vi "Get Connector Pane Info.vi"(8 "error in (no error)":errorcluster, 11 "vi reference":refnum<vi>) -> (0 "error out":errorcluster, 3 "Terminals":T1[](array[typedef]))   [LabVIEW 2025, in "MCP Server.lvlib"]
doc: "Utilizes the Application method \"Get ConPane Datatype\" to read the terminal properties of a subVI without loading it or requiring VI scripting."
uses:
  MCP Server.lvlib
  Terminal.ctl
  <vilib>/Utility/Data Type/NI_Data Type.lvlib
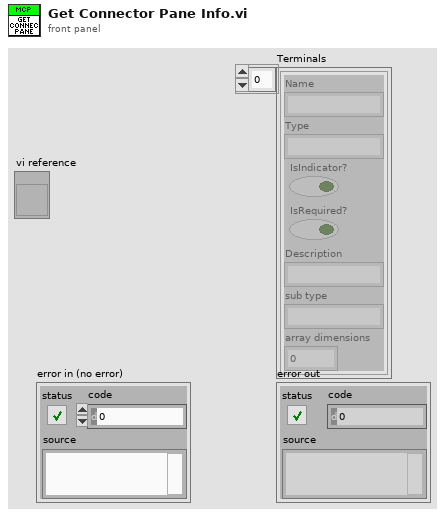
[diagram p1: front panel]
types:
  T1 = typedef "MCP Server.lvlib/Terminal.ctl" = cluster{"Name":string, "Type":string, "IsIndicator?":bool, "IsRequired?":bool, "Description":string, "sub type":string, "array dimensions":i32}
  T2 = typedef "NI_Data Type.lvlib/VI Info.ctl" = cluster{"Connector Pane Pattern":i16, "Connector Pane Rotation":i16, "Flags":u32[], "Modification Date":timestamp, "Asynchronous":bool, "Non-Function":bool, "Subroutine":bool, "SubSystem":bool}
  T3 = typedef "NI_Data Type.lvlib/Data Type.ctl" = enum8{"Invalid Type", "Void", "I8", "I16", "I32", "I64", "U8", "U16", "U32", "U64", "Single Float", "Double Float", "Extended Float", "Single Complex", "Double Complex", "Extended Complex", "Enum U8", "Enum U16", "Enum U32", "Enum U64", "Single Float With Unit", "Double Float With Unit", "Extended Float With Unit", "Single Complex with Unit", "Double Complex with Unit", "Extended Complex with Unit", "Boolean", "String", "Path", "Picture", "Tag", "Array", "Cluster", "Variant", "LV Variant", "Waveform", "Timestamp", "Digital Waveform", "Digital Data", "ExpressData", "Refnum", "External Data", "VI", "Poly VI", "LabVIEW Class Instance", "Fixed Point", "Set Collection", "Map Collection"}
  T4 = typedef "NI_Data Type.lvlib/Memory Info.ctl" = cluster{"Type":T5, "Size":u32}
  T5 = typedef "NI_Data Type.lvlib/Memory Type.ctl" = enum16{"Variable", "Fixed", "Bounded"}
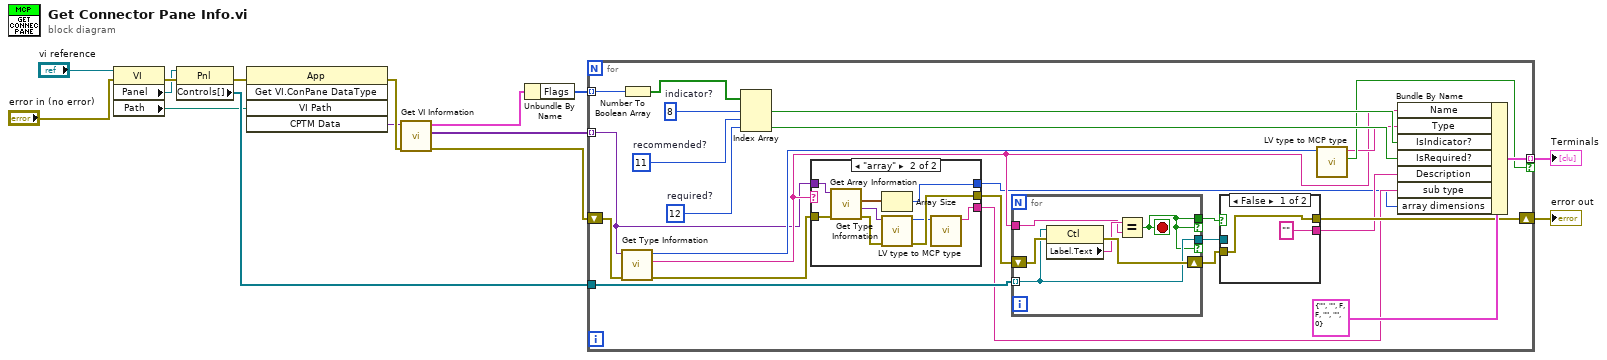
[diagram p0: block diagram]
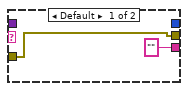
[diagram p2: hidden frame]
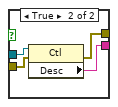
[diagram p3: hidden frame]
diagram:
  n1 = property class="VI"(reference="vi reference", error in="error in (no error)") -> (error out=w6:errorcluster, "Panel"=w4:refnum<vi>, "Path"=w1:path)  [unwired: 1 out]
  n2 = property class="Pnl"(reference=w4, error in=w6) -> (error out=w5:errorcluster, "Controls[]"=w3:refnum<vi>[])  [unwired: 1 out]
  n3 = invoke class="App" method="Get VI.ConPane DataType"(error in=w5, "VI Path"=w1) -> (error out=w12:errorcluster, "CPTM Data"=w8:variant)  [unwired: 3 in, 3 out]
  n4 = call <vilib>:"Get VI Information.vi"("error in (no error)"=w12, "variant"=w8) -> ("error out"=w11:errorcluster, "VI terminal types"=w7:variant[], "VI info"=w9:T2)  [unwired: 6 in, 1 out]
  n5 = Unbundle By Name(w9) -> ("Flags"=w10:u32[])
  n6 = for {
    tunnel: w7 -> [w18] mode=indexing
    tunnel: w10 -> [w39] mode=indexing
    shift-right: [w24] -> w14
    shift-left: w11 -> [w33]
    tunnel: [w29] -> w15 mode=indexing if=w28
    tunnel: w3 -> [w25]
    w35 = 12  # required?
    w36 = 11  # recommended?
    w37 = 8  # indicator?
    n7 = call <vilib>:"Get Type Information.vi"("error in (no error)"=w33, "variant"=w18) -> ("error out"=w34:errorcluster, "name"=w19:string, "type"=w40:T3)  [unwired: 5 in, 2 out]
    n8 = Number To Boolean Array(number=w39) -> (Boolean array=w38:bool[])
    n9 = Index Array(array=w38, index #1=w37, index #2=w36, index #3=w35) -> (element #1=w31:bool, element #3=w30:bool)  [unwired: 1 out]
    n10 = case shown="\"array\"" w19 {
      tunnel: w34 -> [w42 w51]
      tunnel: [w42 w48] -> w20
      tunnel: w18 -> [_ w49]
      tunnel: ["" ("JSON to Insert") w45] -> w17
      tunnel: [_ w43] -> w16
      frame Default {
      }
      frame "array" {
        n11 = call <vilib>:"Get Array Information.vi"("error in (no error)"=w51, "variant"=w49) -> ("error out"=w50:errorcluster, "array element data type"=w47:variant, "array lengths"=w44:T4[])  [unwired: 6 in, 1 out]
        n12 = Array Size(array=w44) -> (size(s)=w43:i32)
        n13 = call <vilib>:"Get Type Information.vi"("error in (no error)"=w50, "variant"=w47) -> ("error out"=w48:errorcluster, "type"=w46:T3)  [unwired: 5 in, 3 out]
        n14 = call "LV type to MCP type.vi"("type"=w46) -> ("JSON to Insert"=w45:string)  [unwired: 9 in, 1 out]
      }
    }
    n15 = for {
      tunnel: w25 -> [w59] mode=indexing
      tunnel: w19 -> [w60]
      shift-right: [w62] -> w26
      shift-left: w20 -> [w63]
      tunnel: [w59] -> w23 if=w58
      tunnel: [w58] -> w21 if=w58
      stop <- w58 stop-if-true
      n16 = property class="Ctl"(reference=w59, error in=w63) -> (error out=w62:errorcluster, "Label.Text"=w61:string)  [unwired: 1 out]
      n17 = Equal?(x=w61, y=w60) -> (x = y?=w58:bool)
    }
    n18 = case shown="False" w21 {
      tunnel: w26 -> [w53 w57]
      tunnel: [w53 w56] -> w24
      tunnel: w23 -> [_ w55]
      tunnel: ["" ("Desc") w54] -> w22
      frame False {
      }
      frame True {
        n19 = property class="Ctl"(reference=w55, error in=w57) -> (error out=w56:errorcluster, "Desc"=w54:string)  [unwired: 1 out]
      }
    }
    n20 = call "LV type to MCP type.vi"("type"=w40) -> ("Valid?"=w28:bool, "JSON to Insert"=w27:string)  [unwired: 9 in]
    n21 = Bundle By Name(cluster=T1 {"Name"="", "Type"="", "IsIndicator?"=FALSE, "IsRequired?"=FALSE, "Description"="", "sub type"="", "array dimensions"=0} ("Terminal"), "Name"=w19, "Type"=w27, "IsIndicator?"=w31, "IsRequired?"=w30, "Description"=w22, "sub type"=w17, "array dimensions"=w16) -> (w29:T1)
  }
  "Terminals" <- w15
  "error out" <- w14
